vi "parse_int16_roslv.vi"   [LabVIEW 2014]
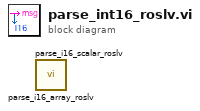
[diagram p0: block diagram]
diagram:
  n1 = call "parse_i16_array_roslv.vi"() -> ()  [unwired: 5 in, 3 out]
  n2 = call "parse_i16_scalar_roslv.vi"() -> ()  [unwired: 5 in, 3 out]
